vi "Last Ack.vi"(7 "Sender":refnum<class "Sender.lvclass">, 10 "Actor":refnum<class "Actor.lvclass">, 11 "Base Actor in":refnum<class "Base Actor.lvclass">) -> (3 "Base Actor out":refnum<class "Base Actor.lvclass">)   [LabVIEW 2021, in "jettl.lvlib" / "Actor.lvlib" / "Base Actor.lvclass"]
uses:
  Base Actor.lvclass
  Actor/Actor.lvclass
  Sender/Sender/Sender.lvclass
  Base Actor.lvclass/Base Actor.ctl
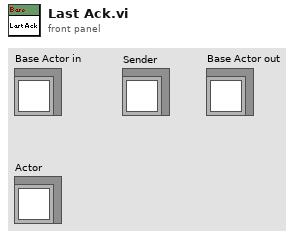
[diagram p1: front panel]
types:
  T1 = typedef "jettl.lvlib/Actor.lvlib/Attributes.ctl" = cluster{"Alias":string, "Address":refnum<user-event>, "Implemented Msgs":T2, "Path":path}
  T2 = typedef "jettl.lvlib/Actor.lvlib/Implemented Msgs.ctl" = set{refnum<class "Msg.lvclass">}
  T3 = typedef "jettl.lvlib/Sender.lvlib/Relation.ctl" = enum16{"Self", "Creator", "Created"}
  T4 = typedef "jettl.lvlib/Actor.lvlib/Alias to Created Attributes.ctl" = map{string, T1}
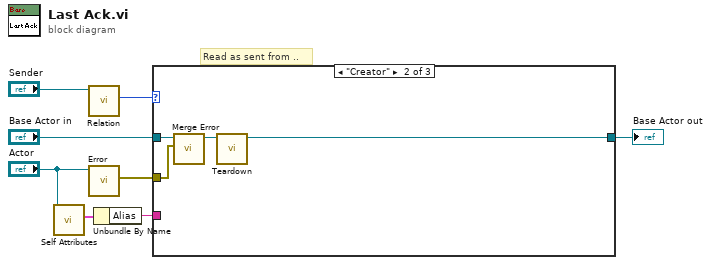
[diagram p0: block diagram]
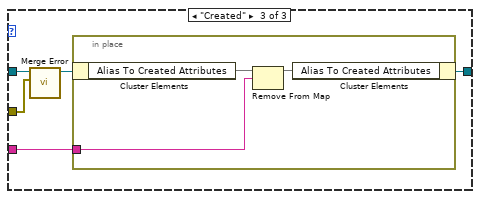
[diagram p3: hidden frame]
diagram:
  # "Read as sent from .."
  n1 = call-dynamic "Self Attributes.vi"("Actor in"="Actor") -> ("Self Attributes"=w3:T1)  [unwired: 10 in]
  n2 = call-dynamic "Relation.vi"("Sender in"="Sender") -> ("Relation"=w5:T3)  [unwired: 10 in]
  n3 = call-dynamic "Error.vi"("Actor in"="Actor") -> ("Error"=w4:errorcluster)  [unwired: 10 in]
  n4 = Unbundle By Name(w3) -> ("Alias"=w2:string)
  n5 = case shown="\"Creator\"" w5 {
    tunnel: "Base Actor in" -> [w9 w10 w17]
    tunnel: [w9 w11 w16] -> w7
    tunnel: w4 -> [_ w13 w15]
    tunnel: w2 -> [_ _ w14]
    frame "Self" {
      # "Case will not fundamentally execute"
    }
    frame "Creator" {
      n6 = call-dynamic "Merge Error.vi"("Error"=w13, "Base Actor in"=w10) -> ("Base Actor out"=w12:refnum<class "Base Actor.lvclass">)  [unwired: 9 in]
      n7 = call-dynamic "Teardown.vi"("Base Actor in"=w12) -> ("Base Actor out"=w11:refnum<class "Base Actor.lvclass">)  [unwired: 10 in]
    }
    frame "Created" {
      n8 = call-dynamic "Merge Error.vi"("Error"=w15, "Base Actor in"=w17) -> ("Base Actor out"=w18:refnum<class "Base Actor.lvclass">)  [unwired: 9 in]
      n9 = in-place {
        in-place-border: w14 -> [w21]
        n10 = in-place-cluster #1(w18) -> ("Alias To Created Attributes"=w20:T4)
        n11 = Remove From Map(10:w21, 11:w20) -> (3:w19:T4)  [unwired: 2 out]
        n12 = in-place-cluster #1("Alias To Created Attributes"=w19) -> (w16:refnum<class "Base Actor.lvclass">)
      }
    }
  }
  "Base Actor out" <- w7
